vi "EventRefTemplate.vi"() -> ()   [LabVIEW 2024, in "AddNewEvent.lvlib"]
uses:
  Event/AddNewEvent.lvlib
panel:
  in  "template":refnum<user-event>
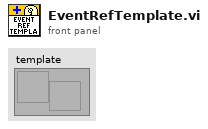
[diagram p1: front panel]
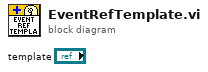
[diagram p0: block diagram]
diagram:
